vi "SigToType.vi"(1 "Sig":string, 2 "Input":T1) -> (0 "Output":T1)   [LabVIEW 2014]
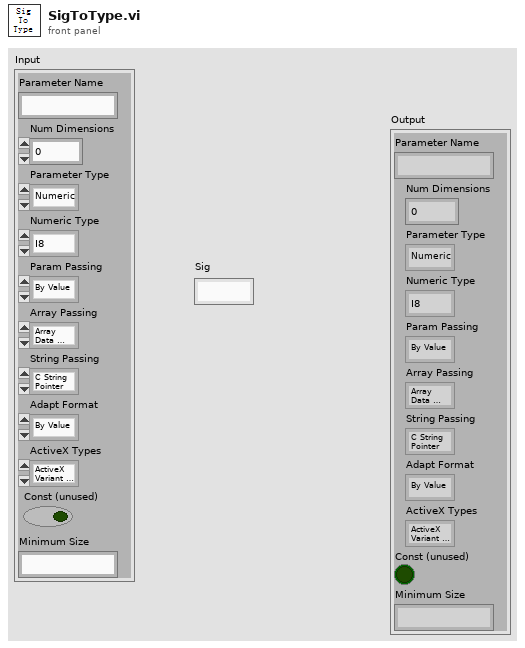
[diagram p1: front panel]
types:
  T1 = cluster{"Parameter Name":string, "Num Dimensions":i32, "Parameter Type":enum16{"Numeric", "Array", "String", "Waveform", "Digital Waveform", "Digital Table", "ActiveX", "Any", "Instance Data Pointer", "Void"}, "Numeric Type":enum16{"I8", "I16", "I32", "I64", "U8", "U16", "U32", "U64", "SGL", "DBL", "PTR INT", "PTR UINT"}, "Param Passing":enum16{"By Value", "Pointer To Value"}, "Array Passing":enum16{"Array Data Pointer", "Array Handle", "Array Handle Pointer"}, "String Passing":enum16{"C String Pointer", "Pascal String Pointer", "String Handle", "String Handle Pointer"}, "Adapt Format":enum16{"By Value", "Pointer To Value"}, "ActiveX Types":enum16{"ActiveX Variant Pointer", "IDispatch* Pointer", "IUnknown* Pointer"}, "Const (unused)":bool, "Minimum Size":string}
  T2 = enum16{"Numeric", "Array", "String", "Waveform", "Digital Waveform", "Digital Table", "ActiveX", "Any", "Instance Data Pointer", "Void"}
  T3 = enum16{"I8", "I16", "I32", "I64", "U8", "U16", "U32", "U64", "SGL", "DBL", "PTR INT", "PTR UINT"}
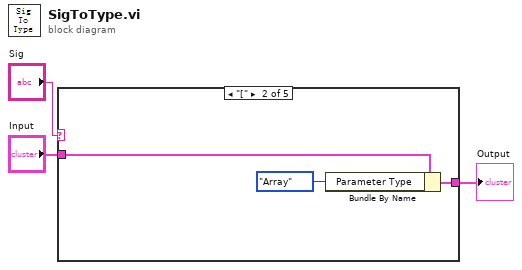
[diagram p0: block diagram]
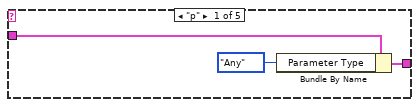
[diagram p2: hidden frame]
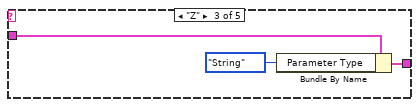
[diagram p3: hidden frame]
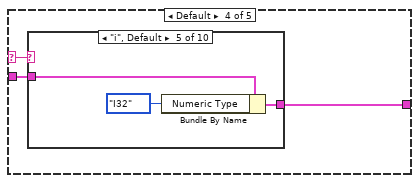
[diagram p4: hidden frame]
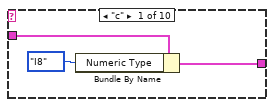
[diagram p5: hidden frame]
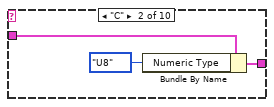
[diagram p6: hidden frame]
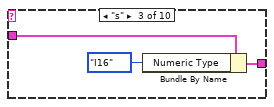
[diagram p7: hidden frame]
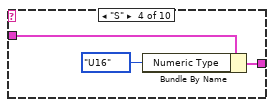
[diagram p8: hidden frame]
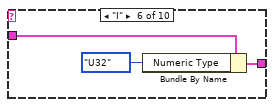
[diagram p9: hidden frame]
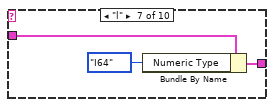
[diagram p10: hidden frame]
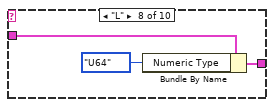
[diagram p11: hidden frame]
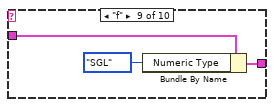
[diagram p12: hidden frame]
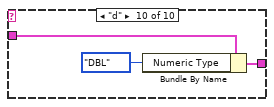
[diagram p13: hidden frame]
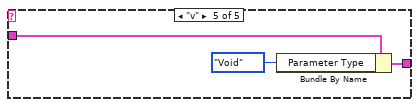
[diagram p14: hidden frame]
diagram:
  n1 = case shown="\"[\"" "Sig" {
    selector: "Sig" -> [_ _ _ w15 _]
    tunnel: "Input" -> [w5 w8 w11 w14 w48]
    tunnel: [w4 w7 w10 w13 w46] -> w1
    frame "p" {
      n2 = Bundle By Name(cluster=w5, "Parameter Type"=T2."Any") -> (w4:T1)
    }
    frame "[" {
      n3 = Bundle By Name(cluster=w8, "Parameter Type"=T2."Array") -> (w7:T1)
    }
    frame "Z" {
      n4 = Bundle By Name(cluster=w11, "Parameter Type"=T2."String") -> (w10:T1)
    }
    frame Default {
      n5 = case shown="\"i\", Default" w15 {
        tunnel: [w17 w19 w22 w26 w28 w31 w34 w37 w40 w43] -> w13
        tunnel: w14 -> [w16 w20 w23 w25 w29 w32 w35 w38 w41 w45]
        frame "c" {
          n6 = Bundle By Name(cluster=w16, "Numeric Type"=T3."I8") -> (w17:T1)
        }
        frame "C" {
          n7 = Bundle By Name(cluster=w20, "Numeric Type"=T3."U8") -> (w19:T1)
        }
        frame "s" {
          n8 = Bundle By Name(cluster=w23, "Numeric Type"=T3."I16") -> (w22:T1)
        }
        frame "S" {
          n9 = Bundle By Name(cluster=w25, "Numeric Type"=T3."U16") -> (w26:T1)
        }
        frame "i", Default {
          n10 = Bundle By Name(cluster=w29, "Numeric Type"=T3."I32") -> (w28:T1)
        }
        frame "I" {
          n11 = Bundle By Name(cluster=w32, "Numeric Type"=T3."U32") -> (w31:T1)
        }
        frame "l" {
          n12 = Bundle By Name(cluster=w35, "Numeric Type"=T3."I64") -> (w34:T1)
        }
        frame "L" {
          n13 = Bundle By Name(cluster=w38, "Numeric Type"=T3."U64") -> (w37:T1)
        }
        frame "f" {
          n14 = Bundle By Name(cluster=w41, "Numeric Type"=T3."SGL") -> (w40:T1)
        }
        frame "d" {
          n15 = Bundle By Name(cluster=w45, "Numeric Type"=T3."DBL") -> (w43:T1)
        }
      }
    }
    frame "v" {
      n16 = Bundle By Name(cluster=w48, "Parameter Type"=T2."Void") -> (w46:T1)
    }
  }
  "Output" <- w1
